vi "New Dispay Settings.vi"(8 "error in (no error)":errorcluster, 10 "Display settings":T1, 11 "IMAQ Display in":refnum<class "HIJ Vision Display.lvclass">) -> (0 "error out":errorcluster, 3 "IMAQ Display out":refnum<class "HIJ Vision Display.lvclass">)   [LabVIEW 2014, in "HIJ Vision Display.lvlib" / "HIJ Vision Display.lvclass"]
uses:
  HIJ Vision Display.lvclass
  DisplaySettings.ctl
  Analyze Parameter/Analyze Parameter Target Point/Target Point.lvclass
  Analyze Parameter/Analyze Parameter Calibration/Analyze Parameter Calibration.lvclass
  HIJ Vision Display.lvclass/HIJ Vision Display.ctl
  Analyze Parameter/Analyze Parameter Calibration/Analyze Parameter Calibration.lvclass/Analyze Parameter Calibration.ctl
  Analyze Parameter/Analyze Parameter Target Point/Target Point.lvclass/Target Point.ctl
  Analyze Actor/Analyze Actor Messages/Set Analyze Parameter Msg/Set Analyze Parameter Msg.lvclass/Set Analyze Parameter Msg.ctl
  <vilib>/ActorFramework/Message Enqueuer/Message Enqueuer.lvclass/Message Enqueuer.ctl
  Analyze Parameter/Analyze Parameter Target Point/Write target point.vi
  Analyze Parameter/Analyze Parameter Calibration/Write Calibration.vi
  <vilib>/ActorFramework/Message Enqueuer/Enqueue.vi
  <vilib>/ActorFramework/Message Priority Queue/Priority Enqueue.vi
  <vilib>/ActorFramework/Message Enqueuer/Message Enqueuer.lvclass
  Analyze Actor/Analyze Actor Messages/Set Analyze Parameter Msg/Set Analyze Parameter Msg.lvclass
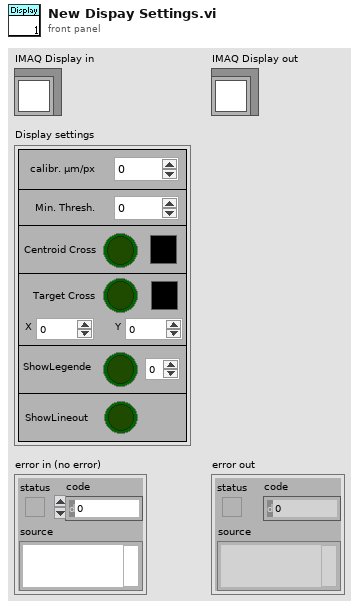
[diagram p1: front panel]
types:
  T1 = typedef "HIJ Vision Display.lvlib/HIJ Vision Display.lvclass/DisplaySettings.ctl" = cluster{"Min. Thresh.":sgl, "X":dbl, "Y":dbl, "ShowLineout":bool, "ScaleParts":i32, "ShowLegende":bool, "Target Cross":bool, "Centroid Cross":bool, "Target color":u32, "Centroid color":u32, "calibr. µm/px":sgl[unit]}
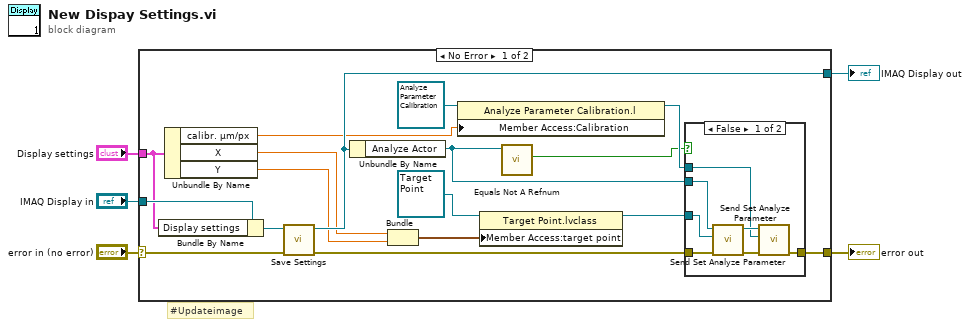
[diagram p0: block diagram]
diagram:
  # "#Updateimage"
  n1 = case shown="No Error" "error in (no error)" {
    selector: "error in (no error)" -> [w20 w32]
    tunnel: [w9 w32] -> w4
    tunnel: [w19 w31] -> w2
    tunnel: "IMAQ Display in" -> [w22 w31]
    tunnel: "Display settings" -> [w17 _]
    frame No Error {
      n2 = Bundle By Name(cluster=w22, "Display settings"=w17) -> (w21:refnum<class "HIJ Vision Display.lvclass">)
      n3 = Unbundle By Name(w17) -> ("calibr. µm/px"=w6:sgl[unit], "X"=w16:dbl, "Y"=w15:dbl)
      n4 = call-dynamic "Save Settings.vi"("error in (no error)"=w20, "IMAQ Display in"=w21) -> ("error out"=w10:errorcluster, "IMAQ Display out"=w19:refnum<class "HIJ Vision Display.lvclass">)  [unwired: 8 in]
      n5 = Unbundle By Name(w19) -> ("Analyze Actor"=w8:refnum<class "Message Enqueuer.lvclass">)
      n6 = Bundle("X"=w16, "Y"=w15) -> (w14:cluster{"X":dbl, "Y":dbl})  [unwired: 1 in]
      n7 = property class="Analyze Parameter Calibration.l"(reference=refnum<class "Analyze Parameter Calibration.lvclass"> refnum ("Analyze Parameter Calibration.lvclass"), "Member Access:Calibration"=w6) -> (reference out=w11:refnum<class "Analyze Parameter Calibration.lvclass">)  [unwired: 1 in, 1 out]
      n8 = property class="Target Point.lvclass"(reference=refnum<class "Target Point.lvclass"> refnum ("Target Point.lvclass"), "Member Access:target point"=w14) -> (reference out=w13:refnum<class "Target Point.lvclass">)  [unwired: 1 in, 1 out]
      n9 = call <vilib>:"Equals Not A Refnum.vi"("Message Enqueuer"=w8) -> ("Not a refnum?"=w7:bool)  [unwired: 10 in]
      n10 = case shown="False" w7 {
        tunnel: w8 -> [w29 _]
        tunnel: w13 -> [w26 _]
        tunnel: w11 -> [w25 _]
        tunnel: w10 -> [w24 w30]
        tunnel: [w23 w30] -> w9
        frame False {
          n11 = call "Send Set Analyze Parameter.vi"("error in (no error)"=w24, "Analyze Parameter"=w26, "Message Enqueuer"=w29) -> ("error out"=w28:errorcluster, "Message Enqueuer out"=w27:refnum<class "Message Enqueuer.lvclass">)  [unwired: 7 in]
          n12 = call "Send Set Analyze Parameter.vi"("error in (no error)"=w28, "Analyze Parameter"=w25, "Message Enqueuer"=w27) -> ("error out"=w23:errorcluster)  [unwired: 7 in, 1 out]
        }
        frame True {
        }
      }
    }
    frame Error {
    }
  }
  "error out" <- w4
  "IMAQ Display out" <- w2
